vi "Add Station Information.vi"(8 "error in (no error)":errorcluster, 10 "Station Info":T1, 11 "ResultProcessor in":refnum<class "ResultProcessor.lvclass">) -> (0 "error out":errorcluster, 3 "ResultProcessor out":refnum<class "ResultProcessor.lvclass">)   [LabVIEW 2015, in "ResultProcessor.lvclass"]
doc: "This VI will add just the station information to the report."
uses:
  ResultProcessor.lvclass
  Report Information/Station Information.ctl
  CommandQueueDataType.ctl
  Report Information/Report Information.lvclass
  Result/Result.lvclass
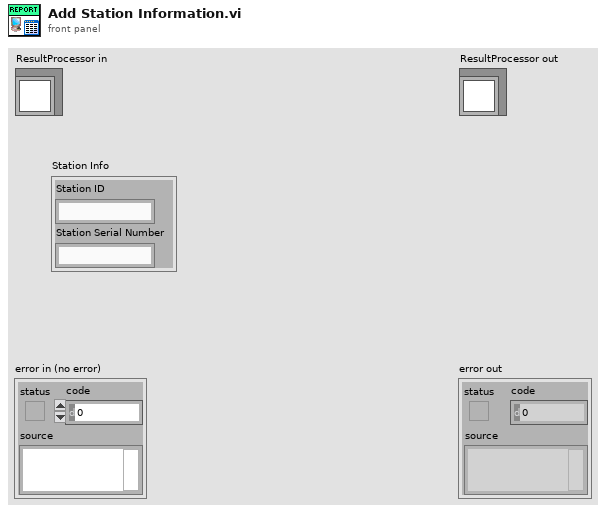
[diagram p1: front panel]
types:
  T1 = typedef "Report Information.lvclass/Station Information.ctl" = cluster{"Station ID":string, "Station Serial Number":string}
  T2 = typedef "ResultProcessor.lvclass/CommandQueueDataType.ctl" = cluster{"Command":enum16{"New Report", "Add Result", "Publish Report", "Shutdown", "Add DUT Information", "Add Station Information", "Add Report Information", "Add Test Information"}, "Report Information.lvclass":refnum<class "Report Information.lvclass">, "Result.lvclass":refnum<class "Result.lvclass">}
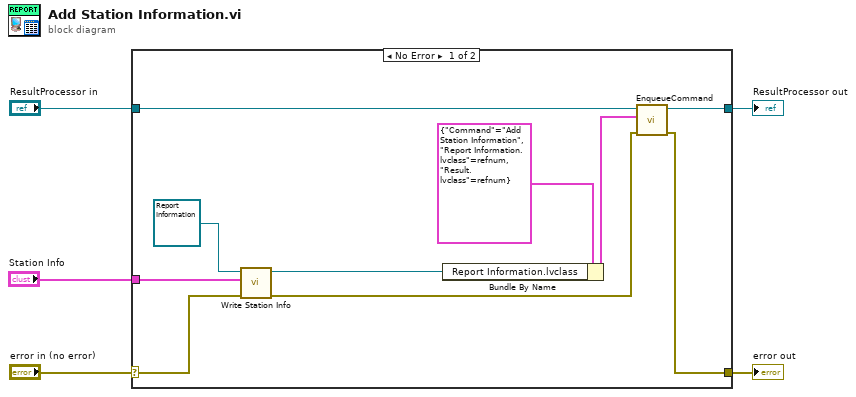
[diagram p0: block diagram]
diagram:
  n1 = case shown="No Error" "error in (no error)" {
    selector: "error in (no error)" -> [w8 w17]
    tunnel: [w13 w17] -> w4
    tunnel: [w14 w16] -> w2
    tunnel: "ResultProcessor in" -> [w15 w16]
    tunnel: "Station Info" -> [w9 _]
    frame No Error {
      n2 = call-dynamic "Write Station Info.vi"("error in (no error)"=w8, "Station Info"=w9, "Report Information in"=refnum<class "Report Information.lvclass"> refnum ("Report Information.lvclass")) -> ("error out"=w7:errorcluster, "Report Information out"=w6:refnum<class "Report Information.lvclass">)  [unwired: 7 in]
      n3 = Bundle By Name(cluster=T2 {"Command"=enum."Add Station Information", "Report Information.lvclass"=refnum, "Result.lvclass"=refnum} ("element"), "Report Information.lvclass"=w6) -> (w11:T2)
      n4 = call "EnqueueCommand.vi"("error in (no error)"=w7, "element"=w11, "ResultProcessor in"=w15) -> ("error out"=w13:errorcluster, "ResultProcessor out"=w14:refnum<class "ResultProcessor.lvclass">)  [unwired: 7 in]
    }
    frame Error {
    }
  }
  "error out" <- w4
  "ResultProcessor out" <- w2
